vi "Begin.vi"(8 "error in":errorcluster) -> (0 "error out":errorcluster)   [LabVIEW 2018]
doc: "Called before other user functions, this VI is expected to open initial I/O refnums, load in file data, and do all program initialization. Notice that the <B>error out</B> terminal is simply used for data flow. Wiring it to other structures or subVIs ensures that this VI runs first."
uses:
  <vilib>/Rock Robotics/WPI/DriverStation/WPI_DriverStationRobotMode2.ctl
  <vilib>/Rock Robotics/WPI/Joystick/WPI_JoystickDeviceEnum.ctl
  <vilib>/Rock Robotics/WPI/ThirdParty/Phoenix-LabVIEW/Motor Controller/Controls/CTRE_Phoenix_MotorControl_NeutralMode.ctl
  <vilib>/Rock Robotics/WPI/Solenoid/WPI_SolenoidChannel.ctl
  <vilib>/Rock Robotics/SystemInterfaces/DIO/FPGA_DIOChannel.ctl
  Robot Global Data.vi
  <vilib>/Rock Robotics/Network Tables/NT Write String Array.vi
  <vilib>/Rock Robotics/WPI/Solenoid/WPI_SolenoidOpenSingle.vi
  <vilib>/Rock Robotics/WPI/Switch/WPI_SwitchOpenLimit.vi
  <vilib>/Rock Robotics/SystemInterfaces/DIO/FPGA_DIOPWMChannel.ctl
  <vilib>/Rock Robotics/WPI/SafetyOutput/WPI_SafetyOutputConfigMenu.ctl
  <vilib>/Rock Robotics/WPI/RobotDrive/WPI_RobotDriveOpen2MotorWithTalon.vi
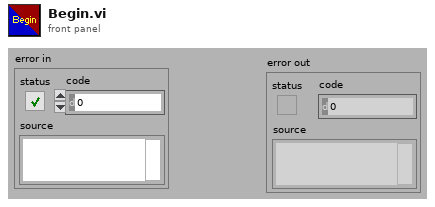
[diagram p1: front panel]
types:
  T1 = enum16{"Idle", "Ground", "Hatch Low", "Hatch Mid", "Hatch High", "Cargo Low", "Cargo Mid", "Cargo High", "Cargo Ship", "Cargo Feed"}
  T2 = typedef "FPGA_DIOChannel.ctl" = enum8{"DIO 0", "DIO 1", "DIO 2", "DIO 3", "DIO 4", "DIO 5", "DIO 6", "DIO 7", "DIO 8", "DIO 9", "DIO MXP 0", "DIO MXP 1", "DIO MXP 2", "DIO MXP 3", "DIO MXP 4", "DIO MXP 5", "DIO MXP 6", "DIO MXP 7", "DIO MXP 8", "DIO MXP 9", "DIO MXP 10", "DIO MXP 11", "DIO MXP 12", "DIO MXP 13", "DIO MXP 14", "DIO MXP 15", "SPI Port CS1", "SPI Port CS2", "SPI Port CS3", "SPI Port MISO", "SPI Port MOSI", "Invalid"}
  T3 = typedef "WPI_SolenoidChannel.ctl" = enum8{"Solenoid 0", "Solenoid 1", "Solenoid 2", "Solenoid 3", "Solenoid 4", "Solenoid 5", "Solenoid 6", "Solenoid 7", "Invalid"}
  T4 = typedef "CTRE_Phoenix_MotorControl_NeutralMode.ctl" = enum8{"EEPROMSetting", "Override to Coast", "Override to Brake"}
  T5 = typedef "WPI_JoystickDeviceEnum.ctl" = enum16{"USB 0", "USB 1", "USB 2", "USB 3", "USB 4", "USB 5"}
  T6 = typedef "WPI_DriverStationRobotMode2.ctl" = enum16{"Autonomous Disabled", "Autonomous Enabled", "Teleop Disabled", "Teleop Enabled", "Disconnected", "Finish", "Test Disabled", "Test Enabled", "Emergency Stopped"}
  T7 = typedef "WPI_SafetyOutputConfigMenu.ctl" = enum16{"Enable", "Disable"}
  T8 = typedef "FPGA_DIOPWMChannel.ctl" = enum8{"PWM 0", "PWM 1", "PWM 2", "PWM 3", "PWM 4", "PWM 5", "PWM 6", "PWM 7", "PWM 8", "PWM 9", "PWM MXP 0", "PWM MXP 1", "PWM MXP 2", "PWM MXP 3", "PWM MXP 4", "PWM MXP 5", "PWM MXP 6", "PWM MXP 7", "PWM MXP 8", "PWM MXP 9", "Invalid"}
  T9 = typedef "WPI_RobotDriveDevRef.ctl" = cluster{"DevStatus":errorcluster, "Motors[]":T10[], "Square Inputs":bool, "Max Output":dbl}
  T10 = typedef "WPI_MotorControlDeviceRef.ctl" = cluster{"DeviceStatus":errorcluster, "Type":T11, "PWM":cluster{"PWM Channel":T8, "DeadBand":T12}, "CAN":cluster{"Device Number":u8, "SetOutput VI Ref":variant, "GetOutput VI Ref":variant, "Enable VI Ref":variant, "Disable VI Ref":variant, "Data":variant}, "Invert":bool, "DIO PWM":cluster{"PWM \"Enable\" Channel":T8, "DIOChannel":T2, "PWM Rate":dbl}}
  T11 = typedef "WPI_MotorControlType.ctl" = enum16{"PWM", "CAN", "DIO PWM"}
  T12 = typedef "WPI_PWMDeadband.ctl" = cluster{"Name":string, "maxPositivePwm":i32, "minPositivePwm":i32, "centerPwm":i32, "maxNegativePwm":i32, "minNegativePwm":i32, "angularRange":u16}
  T13 = typedef "WPI_DigitalInputDevRef.ctl" = cluster{"DevStatus":errorcluster, "DIO Channel":T2}
  T14 = typedef "WPI_JoystickDevRef.ctl" = cluster{"Device":T5}
  T15 = typedef "WPI_SwitchDevRef.ctl" = cluster{"DevStatus":errorcluster, "DIO Channel":T2, "CntIndex":T16, "Normally Closed":bool}
  T16 = typedef "FPGA_CounterCtrSystemIndex.ctl" = enum8{"Ctr 0", "Ctr 1", "Ctr 2", "Ctr 3", "Ctr 4", "Ctr 5", "Ctr 6", "Ctr 7", "Invalid"}
  T17 = typedef "WPI_SolenoidDevRef.ctl" = cluster{"DevStatus":errorcluster, "Pneumatics Control Module":u8, "Forward Solenoid Channel":T3, "Reverse Solenoid Channel":T3}
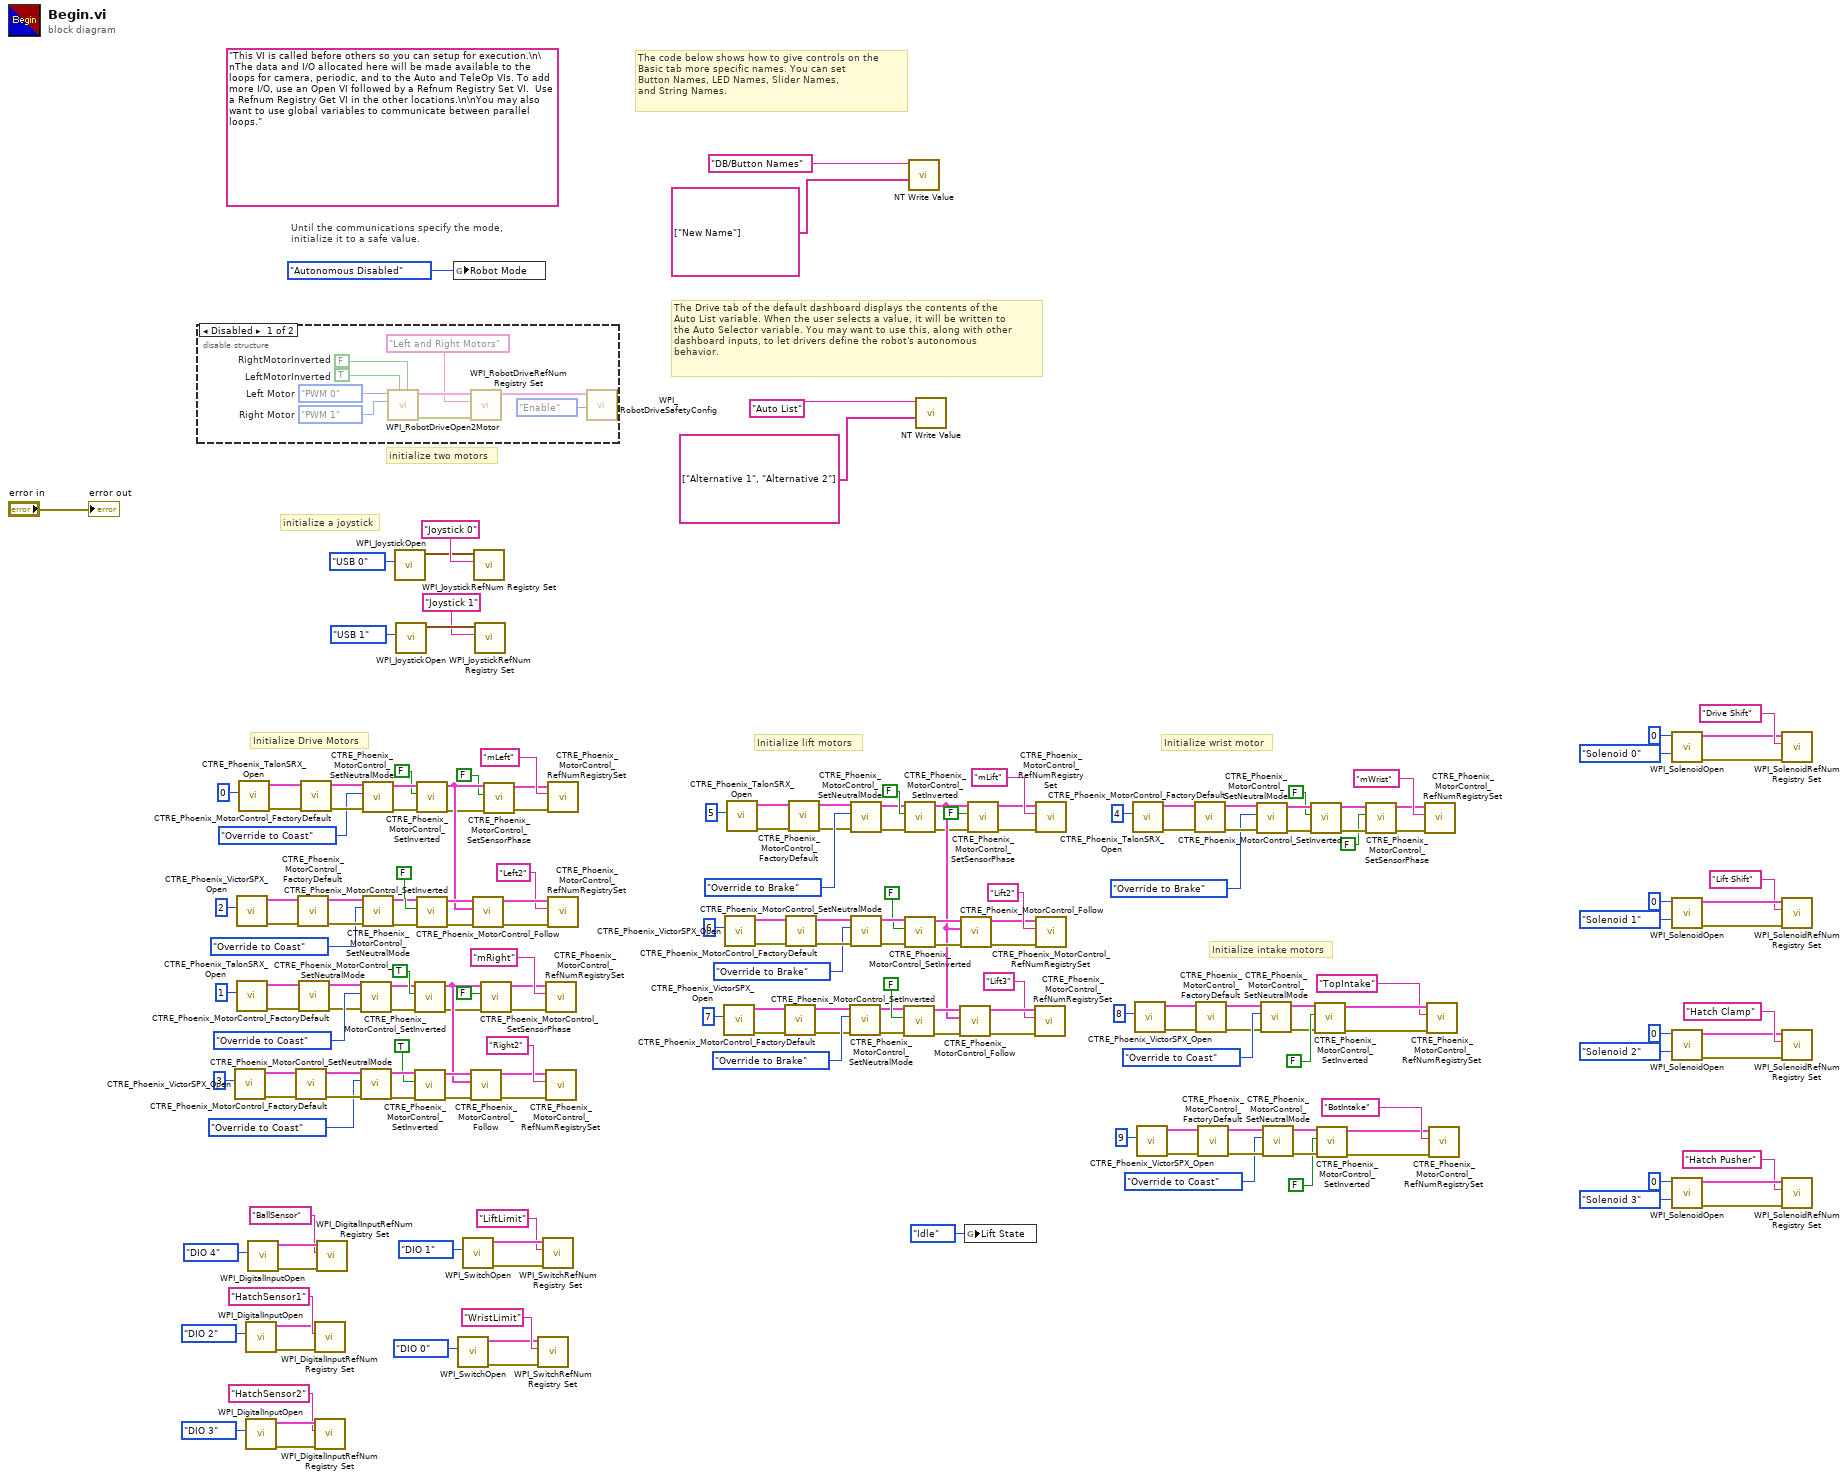
[diagram p0: block diagram]
diagram:
  (unwired) "This VI is called before others so you can setup for execution.\n\nThe data and I/O allocated here will be made available to the loops for camera, periodic, and to the Auto and TeleOp VIs. To add more I/O, use an Open VI followed by a Refnum Registry Set VI.  Use a Refnum Registry Get VI in the other locations.\n\nYou may also want to use global variables to communicate between parallel loops."
  # "Initialize intake motors"
  # "Initialize wrist motor"
  # "Initialize lift motors"
  # "Initialize Drive Motors"
  # "The Drive tab of the default dashboard displays the contents of the\nAuto List variable. When the user selects a value, it will be written to\nthe Auto Selector variable. You may want to use this, along with other\ndashboard inputs, to let drivers define the robot's autonomous\nbehavior."
  # "The code below shows how to give controls on the\nBasic tab more specific names. You can set\nButton Names, LED Names, Slider Names,\nand String Names."
  # "initialize a joystick"
  # "Until the communications specify the mode,\ninitialize it to a safe value."
  # "initialize two motors"
  n1 = disable-structure shown="Disabled" {
    frame Disabled {
      w196 = FPGA_DIOPWMChannel."PWM 1"  # Right Motor
      w197 = FPGA_DIOPWMChannel."PWM 0"  # Left Motor
      w201 = TRUE  # LeftMotorInverted
      w202 = FALSE  # RightMotorInverted
      n2 = call-poly <vilib>:"WPI_RobotDriveOpen2Motor.vi"("Right Motor Inverted"=w202, "Left Motor Inverted"=w201, "Right Motor"=w196, "Left Motor"=w197) -> ("error out"=w198:errorcluster, "RobotDriveDevRef"=w200:T9)  [unwired: 1 in, 5 out]
      n3 = call <vilib>:"WPI_RobotDriveRefNum Registry Set.vi"("error in (no error)"=w198, "refnum name"="Left and Right Motors", "RobotDriveDevRef"=w200) -> ("RobotDriveDevRef"=w195:T9)  [unwired: 1 in, 7 out]
      n4 = call <vilib>:"WPI_RobotDriveSafetyConfig.vi"("mode"=WPI_SafetyOutputConfigMenu."Enable", "RobotDriveDevRef"=w195) -> ()  [unwired: 8 in, 2 out]
    }
    frame Enabled {
    }
  }
  n5 = call <vilib>:"CTRE_Phoenix_VictorSPX_Open.vi"("Device Number"=u8 3) -> ("error out"=w150:errorcluster, "CAN Talon SRX Ref"=w151:T10)  [unwired: 9 in]
  n6 = call <vilib>:"CTRE_Phoenix_VictorSPX_Open.vi"("Device Number"=u8 2) -> ("error out"=w175:errorcluster, "CAN Talon SRX Ref"=w174:T10)  [unwired: 9 in]
  n7 = call <vilib>:"CTRE_Phoenix_TalonSRX_Open.vi"("Device Number"=u8 1) -> ("error out"=w141:errorcluster, "CAN Talon SRX Ref"=w142:T10)  [unwired: 9 in]
  n8 = call <vilib>:"CTRE_Phoenix_TalonSRX_Open.vi"("Device Number"=u8 0) -> ("error out"=w184:errorcluster, "CAN Talon SRX Ref"=w183:T10)  [unwired: 9 in]
  n9 = call <vilib>:"WPI_DigitalInputOpen.vi"("DIO Channel"=FPGA_DIOChannel."DIO 2") -> ("error out"=w16:errorcluster, "DigitalInputDevRef"=w17:T13)  [unwired: 9 in]
  n10 = call <vilib>:"WPI_DigitalInputOpen.vi"("DIO Channel"=FPGA_DIOChannel."DIO 3") -> ("error out"=w15:errorcluster, "DigitalInputDevRef"=w14:T13)  [unwired: 9 in]
  n11 = call <vilib>:"WPI_DigitalInputOpen.vi"("DIO Channel"=FPGA_DIOChannel."DIO 4") -> ("error out"=w21:errorcluster, "DigitalInputDevRef"=w20:T13)  [unwired: 9 in]
  n12 = call <vilib>:"CTRE_Phoenix_MotorControl_FactoryDefault.vi"("error in"=w150, "PhoenixMotorControlDevRef"=w151) -> ("error out"=w152:errorcluster, "PhoenixMotorControlDevRef"=w153:T10)  [unwired: 8 in]
  n13 = call <vilib>:"CTRE_Phoenix_MotorControl_FactoryDefault.vi"("error in"=w175, "PhoenixMotorControlDevRef"=w174) -> ("error out"=w173:errorcluster, "PhoenixMotorControlDevRef"=w172:T10)  [unwired: 8 in]
  n14 = call <vilib>:"CTRE_Phoenix_MotorControl_FactoryDefault.vi"("error in"=w141, "PhoenixMotorControlDevRef"=w142) -> ("error out"=w144:errorcluster, "PhoenixMotorControlDevRef"=w145:T10)  [unwired: 8 in]
  n15 = call <vilib>:"CTRE_Phoenix_MotorControl_FactoryDefault.vi"("error in"=w184, "PhoenixMotorControlDevRef"=w183) -> ("error out"=w181:errorcluster, "PhoenixMotorControlDevRef"=w180:T10)  [unwired: 8 in]
  n16 = call <vilib>:"WPI_DigitalInputRefNum Registry Set.vi"("error in (no error)"=w16, "refnum name"="HatchSensor1", "DigitalInputDevRef"=w17) -> ()  [unwired: 7 in, 2 out]
  n17 = call <vilib>:"WPI_DigitalInputRefNum Registry Set.vi"("error in (no error)"=w15, "refnum name"="HatchSensor2", "DigitalInputDevRef"=w14) -> ()  [unwired: 7 in, 2 out]
  n18 = call <vilib>:"WPI_DigitalInputRefNum Registry Set.vi"("error in (no error)"=w21, "refnum name"="BallSensor", "DigitalInputDevRef"=w20) -> ()  [unwired: 7 in, 2 out]
  n19 = call <vilib>:"CTRE_Phoenix_MotorControl_SetNeutralMode.vi"("error in (no error)"=w144, "Motor Control Neutral Mode"=CTRE_Phoenix_MotorControl_NeutralMode."Override to Coast", "PhoenixMotorControlDevRef"=w145) -> ("error out"=w147:errorcluster, "PhoenixMotorControlDevRef"=w148:T10)  [unwired: 7 in]
  n20 = call <vilib>:"CTRE_Phoenix_MotorControl_SetNeutralMode.vi"("error in (no error)"=w152, "Motor Control Neutral Mode"=CTRE_Phoenix_MotorControl_NeutralMode."Override to Coast", "PhoenixMotorControlDevRef"=w153) -> ("error out"=w76:errorcluster, "PhoenixMotorControlDevRef"=w156:T10)  [unwired: 7 in]
  n21 = call <vilib>:"CTRE_Phoenix_MotorControl_SetNeutralMode.vi"("error in (no error)"=w181, "Motor Control Neutral Mode"=CTRE_Phoenix_MotorControl_NeutralMode."Override to Coast", "PhoenixMotorControlDevRef"=w180) -> ("error out"=w178:errorcluster, "PhoenixMotorControlDevRef"=w177:T10)  [unwired: 7 in]
  n22 = call <vilib>:"CTRE_Phoenix_MotorControl_SetNeutralMode.vi"("error in (no error)"=w173, "Motor Control Neutral Mode"=CTRE_Phoenix_MotorControl_NeutralMode."Override to Coast", "PhoenixMotorControlDevRef"=w172) -> ("error out"=w75:errorcluster, "PhoenixMotorControlDevRef"=w169:T10)  [unwired: 7 in]
  n23 = call <vilib>:"WPI_JoystickOpen.vi"("JoystickDevice"=WPI_JoystickDeviceEnum."USB 0") -> ("JoystickDevRef"=w191:T14)  [unwired: 10 in]
  n24 = call <vilib>:"WPI_JoystickOpen.vi"("JoystickDevice"=WPI_JoystickDeviceEnum."USB 1") -> ("JoystickDevRef"=w137:T14)  [unwired: 10 in]
  n25 = call <vilib>:"CTRE_Phoenix_MotorControl_SetInverted.vi"("error in (no error)"=w147, "Invert?"=TRUE, "PhoenixMotorControlDevRef"=w148) -> ("error out"=w33:errorcluster, "PhoenixMotorControlDevRef"=w36:T10)  [unwired: 7 in]
  n26 = call <vilib>:"CTRE_Phoenix_MotorControl_SetInverted.vi"("error in (no error)"=w76, "Invert?"=TRUE, "PhoenixMotorControlDevRef"=w156) -> ("error out"=w157:errorcluster, "PhoenixMotorControlDevRef"=w158:T10)  [unwired: 7 in]
  n27 = call <vilib>:"CTRE_Phoenix_MotorControl_SetInverted.vi"("error in (no error)"=w178, "Invert?"=FALSE, "PhoenixMotorControlDevRef"=w177) -> ("error out"=w38:errorcluster, "PhoenixMotorControlDevRef"=w41:T10)  [unwired: 7 in]
  n28 = call <vilib>:"CTRE_Phoenix_MotorControl_SetInverted.vi"("error in (no error)"=w75, "Invert?"=FALSE, "PhoenixMotorControlDevRef"=w169) -> ("error out"=w168:errorcluster, "PhoenixMotorControlDevRef"=w167:T10)  [unwired: 7 in]
  n29 = global write "Robot Global Data.vi" "Robot Mode"(WPI_DriverStationRobotMode2."Autonomous Disabled" ("Robot Mode")) -> ()
  n30 = call-poly <vilib>:"WPI_SwitchOpen.vi"("DIO Channel"=FPGA_DIOChannel."DIO 0") -> ("error out"=w3:errorcluster, "SwitchDevRef"=w2:T15)  [unwired: 9 in]
  n31 = call-poly <vilib>:"WPI_SwitchOpen.vi"("DIO Channel"=FPGA_DIOChannel."DIO 1") -> ("error out"=w8:errorcluster, "SwitchDevRef"=w9:T15)  [unwired: 9 in]
  n32 = call <vilib>:"CTRE_Phoenix_MotorControl_Follow.vi"("error in (no error)"=w157, "Master Controller to Follow"=w36, "PhoenixMotorControlDevRef"=w158) -> ("error out"=w159:errorcluster, "PhoenixMotorControlDevRef"=w160:T10)  [unwired: 7 in]
  n33 = call <vilib>:"CTRE_Phoenix_MotorControl_Follow.vi"("error in (no error)"=w168, "Master Controller to Follow"=w41, "PhoenixMotorControlDevRef"=w167) -> ("error out"=w166:errorcluster, "PhoenixMotorControlDevRef"=w165:T10)  [unwired: 7 in]
  n34 = call <vilib>:"WPI_JoystickRefNum Registry Set.vi"("refnum name"="Joystick 0", "JoystickDevRef"=w191) -> ()  [unwired: 8 in, 2 out]
  n35 = call <vilib>:"WPI_JoystickRefNum Registry Set.vi"("refnum name"="Joystick 1", "JoystickDevRef"=w137) -> ()  [unwired: 8 in, 2 out]
  n36 = call <vilib>:"CTRE_Phoenix_MotorControl_SetSensorPhase.vi"("error in (no error)"=w33, "PhaseSensor"=FALSE, "PhoenixMotorControlDevRef"=w36) -> ("error out"=w34:errorcluster, "PhoenixMotorControlDevRef"=w35:T10)  [unwired: 7 in]
  n37 = call <vilib>:"CTRE_Phoenix_MotorControl_SetSensorPhase.vi"("error in (no error)"=w38, "PhaseSensor"=FALSE, "PhoenixMotorControlDevRef"=w41) -> ("error out"=w39:errorcluster, "PhoenixMotorControlDevRef"=w40:T10)  [unwired: 7 in]
  n38 = call <vilib>:"WPI_SwitchRefNum Registry Set.vi"("error in (no error)"=w3, "refnum name"="WristLimit", "SwitchDevRef"=w2) -> ()  [unwired: 7 in, 2 out]
  n39 = call <vilib>:"WPI_SwitchRefNum Registry Set.vi"("error in (no error)"=w8, "refnum name"="LiftLimit", "SwitchDevRef"=w9) -> ()  [unwired: 7 in, 2 out]
  n40 = call <vilib>:"CTRE_Phoenix_MotorControl_RefNumRegistrySet.vi"("error in (no error)"=w34, "refnum name"="mRight", "PhoenixMotorControlDevRef"=w35) -> ()  [unwired: 7 in, 2 out]
  n41 = call <vilib>:"CTRE_Phoenix_MotorControl_RefNumRegistrySet.vi"("error in (no error)"=w159, "refnum name"="Right2", "PhoenixMotorControlDevRef"=w160) -> ()  [unwired: 7 in, 2 out]
  n42 = call <vilib>:"CTRE_Phoenix_MotorControl_RefNumRegistrySet.vi"("error in (no error)"=w39, "refnum name"="mLeft", "PhoenixMotorControlDevRef"=w40) -> ()  [unwired: 7 in, 2 out]
  n43 = call <vilib>:"CTRE_Phoenix_MotorControl_RefNumRegistrySet.vi"("error in (no error)"=w166, "refnum name"="Left2", "PhoenixMotorControlDevRef"=w165) -> ()  [unwired: 7 in, 2 out]
  n44 = call <vilib>:"CTRE_Phoenix_VictorSPX_Open.vi"("Device Number"=u8 7) -> ("error out"=w110:errorcluster, "CAN Talon SRX Ref"=w109:T10)  [unwired: 9 in]
  n45 = call <vilib>:"CTRE_Phoenix_VictorSPX_Open.vi"("Device Number"=u8 6) -> ("error out"=w123:errorcluster, "CAN Talon SRX Ref"=w124:T10)  [unwired: 9 in]
  n46 = call <vilib>:"CTRE_Phoenix_TalonSRX_Open.vi"("Device Number"=u8 5) -> ("error out"=w114:errorcluster, "CAN Talon SRX Ref"=w115:T10)  [unwired: 9 in]
  n47 = call <vilib>:"CTRE_Phoenix_MotorControl_FactoryDefault.vi"("error in"=w110, "PhoenixMotorControlDevRef"=w109) -> ("error out"=w108:errorcluster, "PhoenixMotorControlDevRef"=w107:T10)  [unwired: 8 in]
  n48 = call <vilib>:"CTRE_Phoenix_MotorControl_FactoryDefault.vi"("error in"=w123, "PhoenixMotorControlDevRef"=w124) -> ("error out"=w125:errorcluster, "PhoenixMotorControlDevRef"=w126:T10)  [unwired: 8 in]
  n49 = call <vilib>:"CTRE_Phoenix_MotorControl_FactoryDefault.vi"("error in"=w114, "PhoenixMotorControlDevRef"=w115) -> ("error out"=w117:errorcluster, "PhoenixMotorControlDevRef"=w118:T10)  [unwired: 8 in]
  n50 = call <vilib>:"CTRE_Phoenix_MotorControl_SetNeutralMode.vi"("error in (no error)"=w108, "Motor Control Neutral Mode"=CTRE_Phoenix_MotorControl_NeutralMode."Override to Brake", "PhoenixMotorControlDevRef"=w107) -> ("error out"=w77:errorcluster, "PhoenixMotorControlDevRef"=w105:T10)  [unwired: 7 in]
  n51 = call <vilib>:"CTRE_Phoenix_MotorControl_SetNeutralMode.vi"("error in (no error)"=w117, "Motor Control Neutral Mode"=CTRE_Phoenix_MotorControl_NeutralMode."Override to Brake", "PhoenixMotorControlDevRef"=w118) -> ("error out"=w120:errorcluster, "PhoenixMotorControlDevRef"=w121:T10)  [unwired: 7 in]
  n52 = call <vilib>:"CTRE_Phoenix_MotorControl_SetNeutralMode.vi"("error in (no error)"=w125, "Motor Control Neutral Mode"=CTRE_Phoenix_MotorControl_NeutralMode."Override to Brake", "PhoenixMotorControlDevRef"=w126) -> ("error out"=w78:errorcluster, "PhoenixMotorControlDevRef"=w129:T10)  [unwired: 7 in]
  n53 = call <vilib>:"CTRE_Phoenix_MotorControl_SetInverted.vi"("error in (no error)"=w77, "Invert?"=FALSE, "PhoenixMotorControlDevRef"=w105) -> ("error out"=w104:errorcluster, "PhoenixMotorControlDevRef"=w103:T10)  [unwired: 7 in]
  n54 = call <vilib>:"CTRE_Phoenix_MotorControl_SetInverted.vi"("error in (no error)"=w120, "Invert?"=FALSE, "PhoenixMotorControlDevRef"=w121) -> ("error out"=w28:errorcluster, "PhoenixMotorControlDevRef"=w31:T10)  [unwired: 7 in]
  n55 = call <vilib>:"CTRE_Phoenix_MotorControl_SetInverted.vi"("error in (no error)"=w78, "Invert?"=FALSE, "PhoenixMotorControlDevRef"=w129) -> ("error out"=w130:errorcluster, "PhoenixMotorControlDevRef"=w131:T10)  [unwired: 7 in]
  n56 = call-poly <vilib>:"NT Write Value.vi"("String Array"=string[] ["New Name"], "Name"="DB/Button Names") -> ()  [unwired: 9 in, 1 out]
  n57 = call-poly <vilib>:"NT Write Value.vi"("String Array"=string[] ["Alternative 1", "Alternative 2"], "Name"="Auto List") -> ()  [unwired: 9 in, 1 out]
  n58 = call <vilib>:"CTRE_Phoenix_MotorControl_Follow.vi"("error in (no error)"=w104, "Master Controller to Follow"=w31, "PhoenixMotorControlDevRef"=w103) -> ("error out"=w102:errorcluster, "PhoenixMotorControlDevRef"=w101:T10)  [unwired: 7 in]
  n59 = call <vilib>:"CTRE_Phoenix_MotorControl_Follow.vi"("error in (no error)"=w130, "Master Controller to Follow"=w31, "PhoenixMotorControlDevRef"=w131) -> ("error out"=w132:errorcluster, "PhoenixMotorControlDevRef"=w133:T10)  [unwired: 7 in]
  n60 = global write "Robot Global Data.vi" "Lift State"(T1."Idle" ("Lift State")) -> ()
  n61 = call <vilib>:"CTRE_Phoenix_MotorControl_SetSensorPhase.vi"("error in (no error)"=w28, "PhaseSensor"=FALSE, "PhoenixMotorControlDevRef"=w31) -> ("error out"=w27:errorcluster, "PhoenixMotorControlDevRef"=w30:T10)  [unwired: 7 in]
  n62 = call <vilib>:"CTRE_Phoenix_MotorControl_RefNumRegistrySet.vi"("error in (no error)"=w102, "refnum name"="Lift3", "PhoenixMotorControlDevRef"=w101) -> ()  [unwired: 7 in, 2 out]
  n63 = call <vilib>:"CTRE_Phoenix_MotorControl_RefNumRegistrySet.vi"("error in (no error)"=w27, "refnum name"="mLift", "PhoenixMotorControlDevRef"=w30) -> ()  [unwired: 7 in, 2 out]
  n64 = call <vilib>:"CTRE_Phoenix_MotorControl_RefNumRegistrySet.vi"("error in (no error)"=w132, "refnum name"="Lift2", "PhoenixMotorControlDevRef"=w133) -> ()  [unwired: 7 in, 2 out]
  n65 = call <vilib>:"CTRE_Phoenix_TalonSRX_Open.vi"("Device Number"=u8 4) -> ("error out"=w99:errorcluster, "CAN Talon SRX Ref"=w98:T10)  [unwired: 9 in]
  n66 = call <vilib>:"CTRE_Phoenix_VictorSPX_Open.vi"("Device Number"=u8 8) -> ("error out"=w87:errorcluster, "CAN Talon SRX Ref"=w86:T10)  [unwired: 9 in]
  n67 = call <vilib>:"CTRE_Phoenix_VictorSPX_Open.vi"("Device Number"=u8 9) -> ("error out"=w64:errorcluster, "CAN Talon SRX Ref"=w65:T10)  [unwired: 9 in]
  n68 = call <vilib>:"CTRE_Phoenix_MotorControl_FactoryDefault.vi"("error in"=w99, "PhoenixMotorControlDevRef"=w98) -> ("error out"=w96:errorcluster, "PhoenixMotorControlDevRef"=w95:T10)  [unwired: 8 in]
  n69 = call <vilib>:"CTRE_Phoenix_MotorControl_FactoryDefault.vi"("error in"=w87, "PhoenixMotorControlDevRef"=w86) -> ("error out"=w85:errorcluster, "PhoenixMotorControlDevRef"=w84:T10)  [unwired: 8 in]
  n70 = call <vilib>:"CTRE_Phoenix_MotorControl_FactoryDefault.vi"("error in"=w64, "PhoenixMotorControlDevRef"=w65) -> ("error out"=w66:errorcluster, "PhoenixMotorControlDevRef"=w67:T10)  [unwired: 8 in]
  n71 = call <vilib>:"CTRE_Phoenix_MotorControl_SetNeutralMode.vi"("error in (no error)"=w96, "Motor Control Neutral Mode"=CTRE_Phoenix_MotorControl_NeutralMode."Override to Brake", "PhoenixMotorControlDevRef"=w95) -> ("error out"=w93:errorcluster, "PhoenixMotorControlDevRef"=w92:T10)  [unwired: 7 in]
  n72 = call <vilib>:"CTRE_Phoenix_MotorControl_SetNeutralMode.vi"("error in (no error)"=w85, "Motor Control Neutral Mode"=CTRE_Phoenix_MotorControl_NeutralMode."Override to Coast", "PhoenixMotorControlDevRef"=w84) -> ("error out"=w79:errorcluster, "PhoenixMotorControlDevRef"=w83:T10)  [unwired: 7 in]
  n73 = call <vilib>:"CTRE_Phoenix_MotorControl_SetNeutralMode.vi"("error in (no error)"=w66, "Motor Control Neutral Mode"=CTRE_Phoenix_MotorControl_NeutralMode."Override to Coast", "PhoenixMotorControlDevRef"=w67) -> ("error out"=w72:errorcluster, "PhoenixMotorControlDevRef"=w68:T10)  [unwired: 7 in]
  n74 = call <vilib>:"CTRE_Phoenix_MotorControl_SetInverted.vi"("error in (no error)"=w93, "Invert?"=FALSE, "PhoenixMotorControlDevRef"=w92) -> ("error out"=w26:errorcluster, "PhoenixMotorControlDevRef"=w25:T10)  [unwired: 7 in]
  n75 = call <vilib>:"CTRE_Phoenix_MotorControl_SetInverted.vi"("error in (no error)"=w79, "Invert?"=FALSE, "PhoenixMotorControlDevRef"=w83) -> ("error out"=w82:errorcluster, "PhoenixMotorControlDevRef"=w81:T10)  [unwired: 7 in]
  n76 = call <vilib>:"CTRE_Phoenix_MotorControl_SetInverted.vi"("error in (no error)"=w72, "Invert?"=FALSE, "PhoenixMotorControlDevRef"=w68) -> ("error out"=w69:errorcluster, "PhoenixMotorControlDevRef"=w70:T10)  [unwired: 7 in]
  n77 = call <vilib>:"CTRE_Phoenix_MotorControl_SetSensorPhase.vi"("error in (no error)"=w26, "PhaseSensor"=FALSE, "PhoenixMotorControlDevRef"=w25) -> ("error out"=w23:errorcluster, "PhoenixMotorControlDevRef"=w24:T10)  [unwired: 7 in]
  n78 = call <vilib>:"CTRE_Phoenix_MotorControl_RefNumRegistrySet.vi"("error in (no error)"=w23, "refnum name"="mWrist", "PhoenixMotorControlDevRef"=w24) -> ()  [unwired: 7 in, 2 out]
  n79 = call <vilib>:"CTRE_Phoenix_MotorControl_RefNumRegistrySet.vi"("error in (no error)"=w82, "refnum name"="TopIntake", "PhoenixMotorControlDevRef"=w81) -> ()  [unwired: 7 in, 2 out]
  n80 = call <vilib>:"CTRE_Phoenix_MotorControl_RefNumRegistrySet.vi"("error in (no error)"=w69, "refnum name"="BotIntake", "PhoenixMotorControlDevRef"=w70) -> ()  [unwired: 7 in, 2 out]
  n81 = call-poly <vilib>:"WPI_SolenoidOpen.vi"("Solenoid Channel"=WPI_SolenoidChannel."Solenoid 0", "Pneumatics Control Module (0)"=u8 0) -> ("error out"=w57:errorcluster, "SolenoidDevRef"=w59:T17)  [unwired: 8 in]
  n82 = call-poly <vilib>:"WPI_SolenoidOpen.vi"("Solenoid Channel"=WPI_SolenoidChannel."Solenoid 1", "Pneumatics Control Module (0)"=u8 0) -> ("error out"=w56:errorcluster, "SolenoidDevRef"=w54:T17)  [unwired: 8 in]
  n83 = call-poly <vilib>:"WPI_SolenoidOpen.vi"("Solenoid Channel"=WPI_SolenoidChannel."Solenoid 2", "Pneumatics Control Module (0)"=u8 0) -> ("error out"=w47:errorcluster, "SolenoidDevRef"=w49:T17)  [unwired: 8 in]
  n84 = call-poly <vilib>:"WPI_SolenoidOpen.vi"("Solenoid Channel"=WPI_SolenoidChannel."Solenoid 3", "Pneumatics Control Module (0)"=u8 0) -> ("error out"=w46:errorcluster, "SolenoidDevRef"=w44:T17)  [unwired: 8 in]
  n85 = call <vilib>:"WPI_SolenoidRefNum Registry Set.vi"("error in (no error)"=w57, "refnum name"="Drive Shift", "SolenoidDevRef"=w59) -> ()  [unwired: 7 in, 2 out]
  n86 = call <vilib>:"WPI_SolenoidRefNum Registry Set.vi"("error in (no error)"=w56, "refnum name"="Lift Shift", "SolenoidDevRef"=w54) -> ()  [unwired: 7 in, 2 out]
  n87 = call <vilib>:"WPI_SolenoidRefNum Registry Set.vi"("error in (no error)"=w47, "refnum name"="Hatch Clamp", "SolenoidDevRef"=w49) -> ()  [unwired: 7 in, 2 out]
  n88 = call <vilib>:"WPI_SolenoidRefNum Registry Set.vi"("error in (no error)"=w46, "refnum name"="Hatch Pusher", "SolenoidDevRef"=w44) -> ()  [unwired: 7 in, 2 out]
  "error out" <- "error in"
